vi "CRYUnflatten Acquisition.vi"(11 "Flatten Acquisition":string) -> (0 "Error?":bool=TRUE, 2 "Acquisition":T1={"Mode"=1, "Name"="", "use ch name"=FALSE, "Record Time"=10.0, "hide rec"=FALSE, "hide play"=FALSE, "rec delay"=0.0, "rec pad"=0.0, "dcc units"=0, "sine gen setting"="", "scope_fft setting"="", "voltmeter setting"="", "rta setting"="", "trig offset(sec)"=0.0, "triggered  record"=FALSE, "trig level"=0.0, "trig unit"=0, "trig slop"=FALSE, "trig timeout(sec)"=0.0, "add record"=FALSE, "EQ"=FALSE, "record table"=[], "play table"=[], "trig channel"="", "Help"=""} {"trig unit" format="%.2f"; "trig level" format="%.2f"; "trig offset(sec)" format="%.2f"; "rec delay" format="%.2f"; "rec pad" format="%.2f"; "Record Time" format="%.2f"}, 3 "Header info":T2={"Data type"="Data            ", "Version"=1, "Dimensions"=0})   [LabVIEW 2013]
uses:
  Typedef Control/CRYAcquisition Cluster.ctl
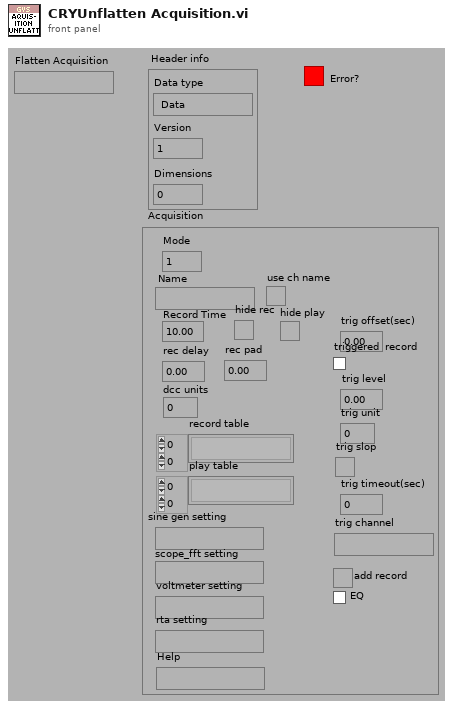
[diagram p1: front panel]
types:
  T1 = typedef "CRYAcquisition Cluster.ctl" = cluster{"Mode":u16, "Name":string, "use ch name":bool, "Record Time":dbl, "hide rec":bool, "hide play":bool, "rec delay":dbl, "rec pad":dbl, "dcc units":i8, "sine gen setting":string, "scope_fft setting":string, "voltmeter setting":string, "rta setting":string, "trig offset(sec)":dbl, "triggered  record":bool, "trig level":dbl, "trig unit":u8, "trig slop":bool, "trig timeout(sec)":dbl, "add record":bool, "EQ":bool, "record table":string[][], "play table":string[][], "trig channel":string, "Help":string}
  T2 = cluster{"Data type":string, "Version":u16, "Dimensions":u8}
  T3 = cluster{"unsigned byte array[0]":u8, "unsigned byte array[1]":u8, "unsigned byte array[2]":u8}
  T4 = cluster{"Mode":u16, "Name":string, "use ch name":bool, "Record Time":dbl, "hide rec":bool, "hide play":bool, "rec delay":dbl, "rec pad":dbl, "dcc units":i8, "sine gen setting":string, "scope_fft setting":string, "voltmeter setting":string, "rta setting":string, "trig offset(sec)":dbl, "triggered  record":bool, "trig level":dbl, "trig unit":u8, "trig slop":bool, "trig timeout(sec)":dbl, "add record":bool, "EQ":bool, "record table":string[][], "play table":string[][]}
  T5 = cluster{"Mode":u16, "Name":string, "use ch name":bool, "Record Time":dbl, "hide rec":bool, "hide play":bool, "rec delay":dbl, "rec pad":dbl, "dcc units":i8, "sine gen setting":string, "scope_fft setting":string, "voltmeter setting":string, "rta setting":string, "trig offset(sec)":dbl, "triggered  record":bool, "trig level":dbl, "trig unit":u8, "trig slop":bool, "trig timeout(sec)":dbl, "add record":bool, "EQ":bool, "record table":string[][], "play table":string[][], "trig channel":string}
  T6 = cluster{"substring":string, u16, "unsigned byte array[2]":u8}
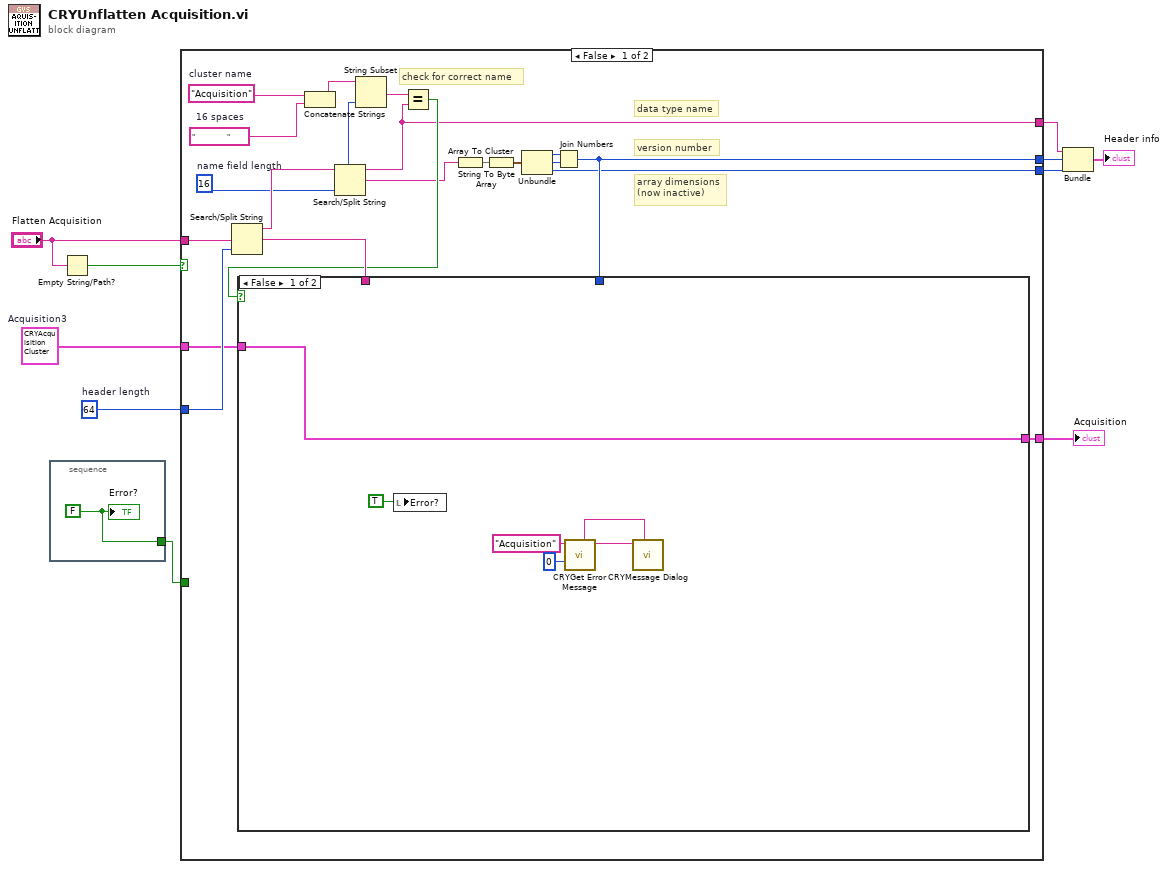
[diagram p0: block diagram]
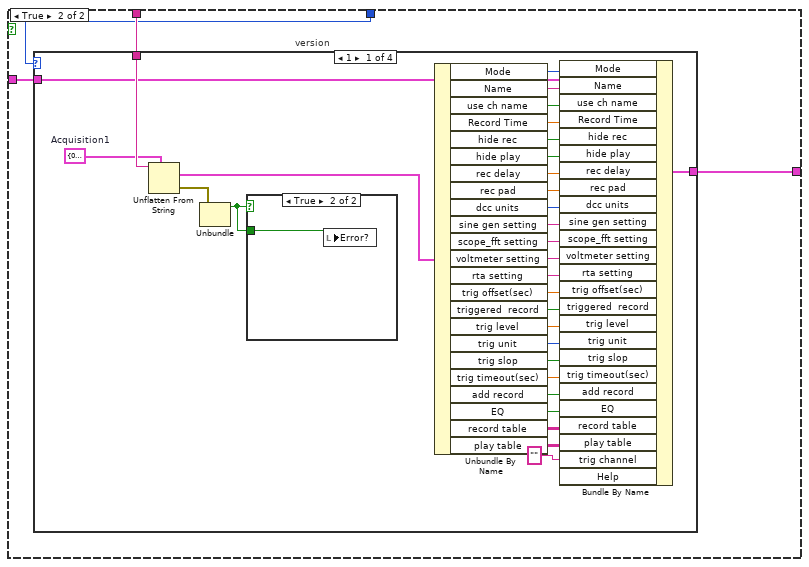
[diagram p2: hidden frame]
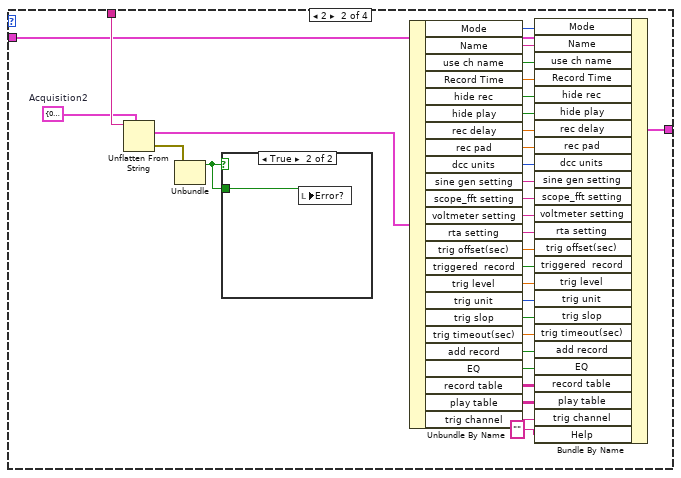
[diagram p4: hidden frame]
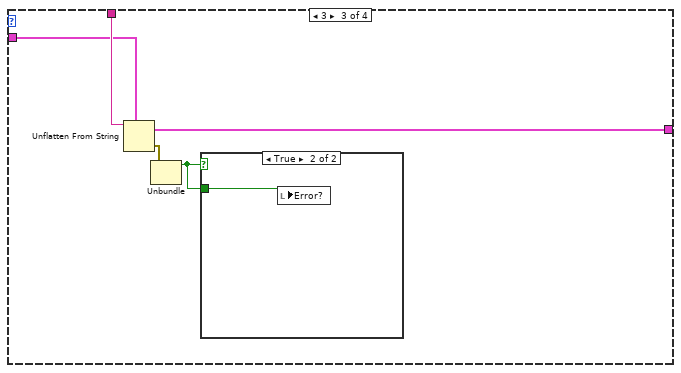
[diagram p6: hidden frame]
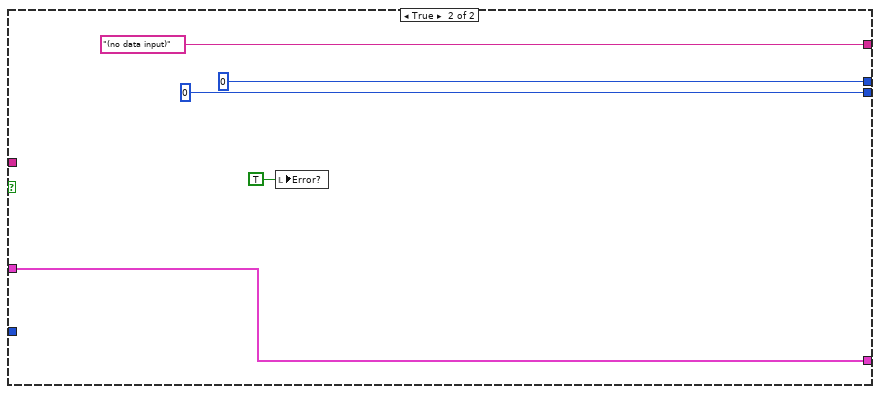
[diagram p9: hidden frame]
diagram:
  w2 = T1 {"Mode"=0, "Name"="", "use ch name"=FALSE, "Record Time"=0.0, "hide rec"=FALSE, "hide play"=FALSE, "rec delay"=0.0, "rec pad"=0.0, "dcc units"=0, "sine gen setting"="", "scope_fft setting"="", "voltmeter setting"="", "rta setting"="", "trig offset(sec)"=0.0, "triggered  record"=FALSE, "trig level"=0.0, "trig unit"=0, "trig slop"=FALSE, "trig timeout(sec)"=0.0, "add record"=FALSE, "EQ"=FALSE, "record table"=[], "play table"=[], "trig channel"="", "Help"=""}  # Acquisition3
  w8 = 64  # header length
  n1 = stacked-sequence {
    tunnel: [w11] -> w3
    frame #0 {
      w11 = FALSE
      "Error?" <- w11
    }
  }
  n2 = Empty String/Path?(string/path="Flatten Acquisition") -> (empty?=w9:bool)
  n3 = case shown="False" w9 {
    tunnel: "Flatten Acquisition" -> [w31 _]
    tunnel: w8 -> [w25 _]
    tunnel: [w22 u16 0] -> w6
    tunnel: [w14 u8 0] -> w7
    tunnel: [w15 "(no data input)" ("substring")] -> w5
    tunnel: w3 -> [_ _]
    tunnel: [w13 w114] -> w1
    tunnel: w2 -> [w12 w114]
    frame False {
      w19 = "                "  # 16 spaces
      w20 = "Acquisition"  # cluster name
      w17 = 16  # name field length
      # "check for correct name"
      # "array dimensions\n(now inactive)"
      # "version number"
      # "data type name"
      n4 = Search/Split String(string=w31, offset (0)=w25) -> (substring before match=w24:string, match + rest of string=w26:string)  [unwired: 2 out]
      n5 = Concatenate Strings(w20, w19) -> (w18:string)
      n6 = Search/Split String(string=w24, offset (0)=w17) -> (substring before match=w15:string, match + rest of string=w21:string)  [unwired: 2 out]
      n7 = String Subset(string=w18, length (rest)=w17) -> (substring=w16:string)  [unwired: 1 out]
      n8 = Equal?(x=w16, y=w15) -> (x = y?=w23:bool)
      n9 = String To Byte Array(string=w21) -> (unsigned byte array=w30:u8[])
      n10 = Array To Cluster(array=w30) -> (cluster=w29:T3)
      n11 = Unbundle(w29) -> ("unsigned byte array[0]"=w28:u8, "unsigned byte array[1]"=w27:u8, "unsigned byte array[2]"=w14:u8)
      n12 = Join Numbers(hi=w28, lo=w27) -> ((hi.lo)=w22:u16)
      n13 = case shown="False" w23 {
        tunnel: w26 -> [_ w41]
        tunnel: w22 -> [_ w40]
        tunnel: [w36 w39] -> w13
        tunnel: w12 -> [w36 w38]
        frame False {
          n14 = local write "Error?"(TRUE) -> ()
          n15 = call "CRYGet Error Message.vi"("Error No"=0, "Kind"="Acquisition") -> ("Message"=w33:string, "Window Title"=w32:string)  [unwired: 4 in, 4 out]
          n16 = call "CRYMessage Dialog.vi"("Window Title"=w32, "Message Content"=w33) -> ()  [unwired: 8 in, 2 out]
        }
        frame True {
          n17 = case "version" shown="1" w40 {
            tunnel: w41 -> [w72 w105 w111 _]
            tunnel: [w67 w101 w107 w113] -> w39
            tunnel: w38 -> [w68 w102 w108 w113]
            frame 1 {
              w42 = "" ("trig channel")
              w69 = T4 {"Mode"=0, "Name"="", "use ch name"=FALSE, "Record Time"=0.0, "hide rec"=FALSE, "hide play"=FALSE, "rec delay"=0.0, "rec pad"=0.0, "dcc units"=0, "sine gen setting"="", "scope_fft setting"="", "voltmeter setting"="", "rta setting"="", "trig offset(sec)"=0.0, "triggered  record"=FALSE, "trig level"=0.0, "trig unit"=0, "trig slop"=FALSE, "trig timeout(sec)"=0.0, "add record"=FALSE, "EQ"=FALSE, "record table"=[], "play table"=[]}  # Acquisition1
              n18 = Unflatten From String(type=w69, binary string=w72) -> (value=w66:T4, error out=w70:errorcluster)  [unwired: 1 in, 3 out]
              n19 = Unbundle(w70) -> ("status"=w71:bool)  [unwired: 2 out]
              n20 = case shown="True" w71 {
                tunnel: w71 -> [_ w73]
                frame False {
                }
                frame True {
                  n21 = local write "Error?"(w73) -> ()
                }
              }
              n22 = Unbundle By Name(w66) -> ("Mode"=w65:u16, "Name"=w64:string, "use ch name"=w63:bool, "Record Time"=w62:dbl, "hide rec"=w61:bool, "hide play"=w60:bool, "rec delay"=w59:dbl, "rec pad"=w58:dbl, "dcc units"=w57:i8, "sine gen setting"=w56:string, "scope_fft setting"=w55:string, "voltmeter setting"=w54:string, "rta setting"=w53:string, "trig offset(sec)"=w52:dbl, "triggered  record"=w51:bool, "trig level"=w50:dbl, "trig unit"=w49:u8, "trig slop"=w48:bool, "trig timeout(sec)"=w47:dbl, "add record"=w46:bool, "EQ"=w45:bool, "record table"=w44:string[][], "play table"=w43:string[][])
              n23 = Bundle By Name(cluster=w68, "Mode"=w65, "Name"=w64, "use ch name"=w63, "Record Time"=w62, "hide rec"=w61, "hide play"=w60, "rec delay"=w59, "rec pad"=w58, "dcc units"=w57, "sine gen setting"=w56, "scope_fft setting"=w55, "voltmeter setting"=w54, "rta setting"=w53, "trig offset(sec)"=w52, "triggered  record"=w51, "trig level"=w50, "trig unit"=w49, "trig slop"=w48, "trig timeout(sec)"=w47, "add record"=w46, "EQ"=w45, "record table"=w44, "play table"=w43, "trig channel"=w42, "Help"=w42) -> (w67:T1)
            }
            frame 2 {
              w76 = T5 {"Mode"=0, "Name"="", "use ch name"=FALSE, "Record Time"=0.0, "hide rec"=FALSE, "hide play"=FALSE, "rec delay"=0.0, "rec pad"=0.0, "dcc units"=0, "sine gen setting"="", "scope_fft setting"="", "voltmeter setting"="", "rta setting"="", "trig offset(sec)"=0.0, "triggered  record"=FALSE, "trig level"=0.0, "trig unit"=0, "trig slop"=FALSE, "trig timeout(sec)"=0.0, "add record"=FALSE, "EQ"=FALSE, "record table"=[], "play table"=[], "trig channel"=""}  # Acquisition2
              n24 = Unflatten From String(type=w76, binary string=w105) -> (value=w100:T5, error out=w103:errorcluster)  [unwired: 1 in, 3 out]
              n25 = Unbundle(w103) -> ("status"=w104:bool)  [unwired: 2 out]
              n26 = case shown="True" w104 {
                tunnel: w104 -> [_ w106]
                frame False {
                }
                frame True {
                  n27 = local write "Error?"(w106) -> ()
                }
              }
              n28 = Unbundle By Name(w100) -> ("Mode"=w99:u16, "Name"=w98:string, "use ch name"=w97:bool, "Record Time"=w96:dbl, "hide rec"=w95:bool, "hide play"=w94:bool, "rec delay"=w93:dbl, "rec pad"=w92:dbl, "dcc units"=w91:i8, "sine gen setting"=w90:string, "scope_fft setting"=w89:string, "voltmeter setting"=w88:string, "rta setting"=w87:string, "trig offset(sec)"=w86:dbl, "triggered  record"=w85:bool, "trig level"=w84:dbl, "trig unit"=w83:u8, "trig slop"=w82:bool, "trig timeout(sec)"=w81:dbl, "add record"=w80:bool, "EQ"=w79:bool, "record table"=w78:string[][], "play table"=w77:string[][], "trig channel"=w75:string)
              n29 = Bundle By Name(cluster=w102, "Mode"=w99, "Name"=w98, "use ch name"=w97, "Record Time"=w96, "hide rec"=w95, "hide play"=w94, "rec delay"=w93, "rec pad"=w92, "dcc units"=w91, "sine gen setting"=w90, "scope_fft setting"=w89, "voltmeter setting"=w88, "rta setting"=w87, "trig offset(sec)"=w86, "triggered  record"=w85, "trig level"=w84, "trig unit"=w83, "trig slop"=w82, "trig timeout(sec)"=w81, "add record"=w80, "EQ"=w79, "record table"=w78, "play table"=w77, "trig channel"=w75, "Help"="" ("trig channel")) -> (w101:T1)
            }
            frame 3 {
              n30 = Unflatten From String(type=w108, binary string=w111) -> (value=w107:T1, error out=w109:errorcluster)  [unwired: 1 in, 3 out]
              n31 = Unbundle(w109) -> ("status"=w110:bool)  [unwired: 2 out]
              n32 = case shown="True" w110 {
                tunnel: w110 -> [_ w112]
                frame False {
                }
                frame True {
                  n33 = local write "Error?"(w112) -> ()
                }
              }
            }
            frame Default {
            }
          }
        }
      }
    }
    frame True {
      n34 = local write "Error?"(TRUE ("Error?")) -> ()
    }
  }
  "Acquisition" <- w1
  n35 = Bundle("substring"=w5, w6, "unsigned byte array[2]"=w7) -> (→"Header info":T6)  [unwired: 1 out]
